vi "Outside.vi"(10 "Current_char":string, 11 "Accumulator":refnum<class "Accumulator.lvclass">) -> (2 "End?":bool, 3 "Accumulator'":refnum<class "Accumulator.lvclass">)   [LabVIEW 2020, in "Accumulator.lvclass"]
uses:
  Accumulator.lvclass
  Accumulator.lvclass/Accumulator.ctl
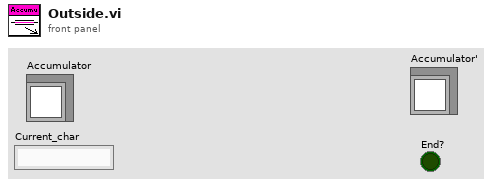
[diagram p1: front panel]
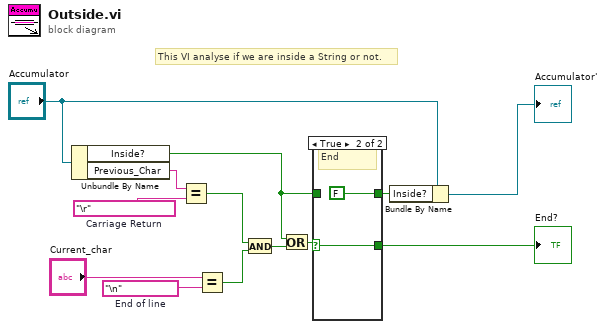
[diagram p0: block diagram]
diagram:
  w6 = "\r"  # Carriage Return
  w8 = "\n"  # End of line
  # "This VI analyse if we are inside a String or not."
  n1 = Unbundle By Name("Accumulator") -> ("Inside?"=w1:bool, "Previous_Char"=w7:string)
  n2 = Equal?(x=w7, y=w6) -> (x = y?=w5:bool)
  n3 = Equal?(x="Current_char", y=w8) -> (x = y?=w11:bool)
  n4 = And(x=w5, y=w11) -> (x .and. y?=w9:bool)
  n5 = Or(x=w1, y=w9) -> (x .or. y?=w4:bool)
  n6 = case shown="True" w4 {
    selector: w4 -> [w15 w16]
    tunnel: [w14 FALSE] -> w3
    tunnel: [w15 w16] -> w2
    tunnel: w1 -> [w14 _]
    frame False {
      # "Continue"
    }
    frame True {
      # "End"
    }
  }
  "End?" <- w2
  n7 = Bundle By Name(cluster="Accumulator", "Inside?"=w3) -> (→"Accumulator'":refnum<class "Accumulator.lvclass">)
